vi "读写行DEMO.vi"() -> ()   [LabVIEW 2012]
panel:
  out "NewLine":string
  out "行读取":string
  in  "停止":bool
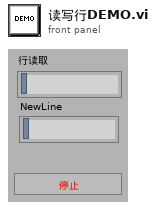
[diagram p1: front panel]
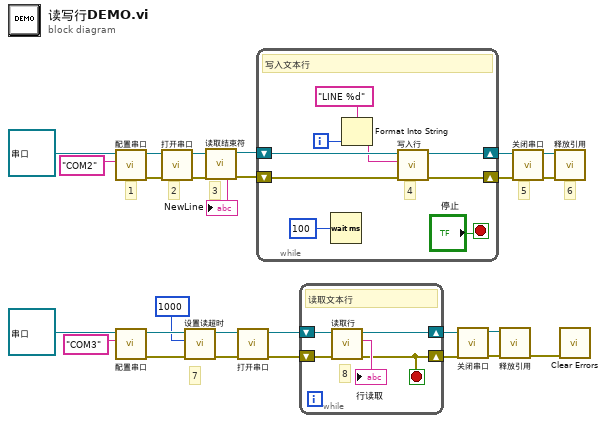
[diagram p0: block diagram]
diagram:
  # "7"
  # "6"
  # "5"
  # "3"
  # "2"
  # "1"
  n1 = call "配置串口.vi"("Port Name"="COM2", "COM 输入"=refnum<class "串口.lvclass"> refnum ("串口.lvclass")) -> ("error out"=w24:errorcluster, "COM 输出"=w25:refnum<class "串口.lvclass">)  [unwired: 8 in]
  n2 = call "配置串口.vi"("Port Name"="COM3", "COM 输入"=refnum<class "串口.lvclass"> refnum ("串口.lvclass")) -> ("error out"=w12:errorcluster, "COM 输出"=w13:refnum<class "串口.lvclass">)  [unwired: 8 in]
  n3 = call "打开串口.vi"("error in (no error)"=w24, "串口 输入"=w25) -> ("error out"=w5:errorcluster, "串口 输出"=w6:refnum<class "串口.lvclass">)  [unwired: 8 in]
  n4 = call "设置读超时.vi"("error in (no error)"=w12, "ReadTimeout"=1000, "串口 输入"=w13) -> ("error out"=w10:errorcluster, "串口 输出"=w11:refnum<class "串口.lvclass">)  [unwired: 7 in]
  n5 = call "读取结束符.vi"("error in (no error)"=w5, "串口 输入"=w6) -> ("error out"=w3:errorcluster, "NewLine"=→"NewLine":string, "串口 输出"=w4:refnum<class "串口.lvclass">)  [unwired: 7 in]
  n6 = call "打开串口.vi"("error in (no error)"=w10, "串口 输入"=w11) -> ("error out"=w14:errorcluster, "串口 输出"=w15:refnum<class "串口.lvclass">)  [unwired: 8 in]
  n7 = while "While循环" {
    shift-right: [w33] -> w22
    shift-left: w3 -> [w35]
    shift-right: [w32] -> w23
    shift-left: w4 -> [w36]
    i -> [w31]
    stop <- "停止" stop-if-true
    # "4"
    # "写入文本行"
    n8 = Wait (ms)(milliseconds to wait=u32 100 ("等待时间（毫秒）")) -> ()  [unwired: 1 out]
    n9 = Format Into String(format string="LINE %d" ("格式字符串"), w31) -> (resulting string=w28:string)  [unwired: 2 in, 1 out]
    n10 = call "写入行.vi"("error in (no error)"=w35, "行数据"=w28, "串口 输入"=w36) -> ("error out"=w33:errorcluster, "串口 输出"=w32:refnum<class "串口.lvclass">)  [unwired: 7 in]
  }
  n11 = while {
    shift-right: [w38] -> w7
    shift-left: w14 -> [w40]
    shift-right: [w37] -> w8
    shift-left: w15 -> [w41]
    stop <- w38 stop-if-true
    # "8"
    # "读取文本行"
    n12 = call "读取行.vi"("error in (no error)"=w40, "串口 输入"=w41) -> ("error out"=w38:errorcluster, "行读取"=→"行读取":string, "串口 输出"=w37:refnum<class "串口.lvclass">)  [unwired: 7 in]
  }
  n13 = call "关闭串口.vi"("error in (no error)"=w7, "串口 输入"=w8) -> ("error out"=w16:errorcluster, "串口 输出"=w17:refnum<class "串口.lvclass">)  [unwired: 8 in]
  n14 = call "释放引用.vi"("error in (no error)"=w16, "串口 输入"=w17) -> ("error out"=w1:errorcluster)  [unwired: 8 in, 1 out]
  n15 = call "关闭串口.vi"("error in (no error)"=w22, "串口 输入"=w23) -> ("error out"=w21:errorcluster, "串口 输出"=w20:refnum<class "串口.lvclass">)  [unwired: 8 in]
  n16 = call "释放引用.vi"("error in (no error)"=w21, "串口 输入"=w20) -> ()  [unwired: 8 in, 2 out]
  n17 = call <vilib>:"Clear Errors.vi"("error in (no error)"=w1) -> ()  [unwired: 6 in, 1 out]
